vi "RenderClear.vi"(8 "No Error":errorcluster, 11 "Renderer [SDL_Renderer *]":i64 format="%.0x") -> (0 "error out":errorcluster)   [LabVIEW 2026, in "SDL3.lvlib" / "Render.lvlib"]
doc: "<B>Summary</B>\nClear the current rendering target with the drawing color.\n\n<B>Remarks</B>\nThis function clears the entire rendering target, ignoring the viewport and the clip rectangle. Note, that clearing will also set/fill all pixels of the rendering target to current renderer draw color, so make sure to invoke SDL_SetRenderDrawColor() when needed."
uses:
  Render.lvlib
  <vilib>/Utility/error.llb/Error Cluster From Error Code.vi
  Error/Error.lvlib
  Lib/SDL3.dll
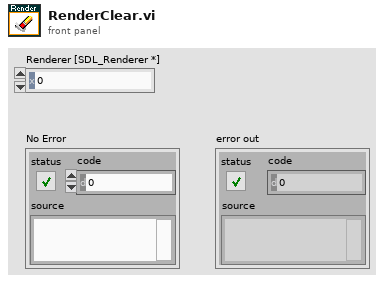
[diagram p1: front panel]
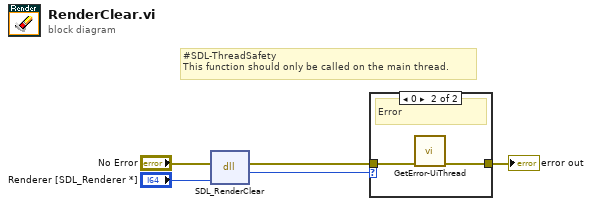
[diagram p0: block diagram]
diagram:
  # "#SDL-ThreadSafety\nThis function should only be called on the main thread."
  n1 = dll-call lib="C:/Users/saukko/Dev/LV-SDL3/Sources/SDL3/Lib/SDL3.*" fn="SDL_RenderClear"(error in="No Error", "renderer"="Renderer [SDL_Renderer *]") -> (error out=w2:errorcluster, "return type"=w1:i32)  [unwired: 3 in, 1 out]
  n2 = case shown="0" w1 {
    tunnel: w2 -> [w6 w8]
    tunnel: [w6 w7] -> w4
    frame Default {
      # "Ok"
    }
    frame 0 {
      # "Error"
      n3 = call "GetError-UiThread.vi"("No Error"=w8) -> ("error out"=w7:errorcluster)  [unwired: 10 in]
    }
  }
  "error out" <- w4
